vi "S101_ACT2ndCtrl.vi"(0 "SI101_AverageReactorCoolantTemperature.lvclass":refnum<class "SI101_AverageReactorCoolantTemperature.lvclass">, 1 "ACT Loop1":dbl, 2 "ACT Loop2":dbl, 3 "ACT Loop3":dbl, 4 "ACT Loop4":dbl, 5 "error in (no error)":errorcluster, 8 "APs":cluster{"AP1":dbl, "AP2":dbl, "AP3":dbl}) -> (14 "SI101_AverageReactorCoolantTemperature.lvclass out":refnum<class "SI101_AverageReactorCoolantTemperature.lvclass">, 15 "ACT 2nd Ctrl":dbl, 16 "ACT D-Comp":dbl, 17 "ACT 2ND MAX LIM":dbl, 19 "error IO":errorcluster)   [LabVIEW 2022 SP3, in "SI101_AverageReactorCoolantTemperature.lvclass"]
uses:
  SI101_AverageReactorCoolantTemperature.lvclass
  SI101_AverageReactorCoolantTemperature.lvclass/SI101_AverageReactorCoolantTemperature.ctl
panel:
  # "SI101"
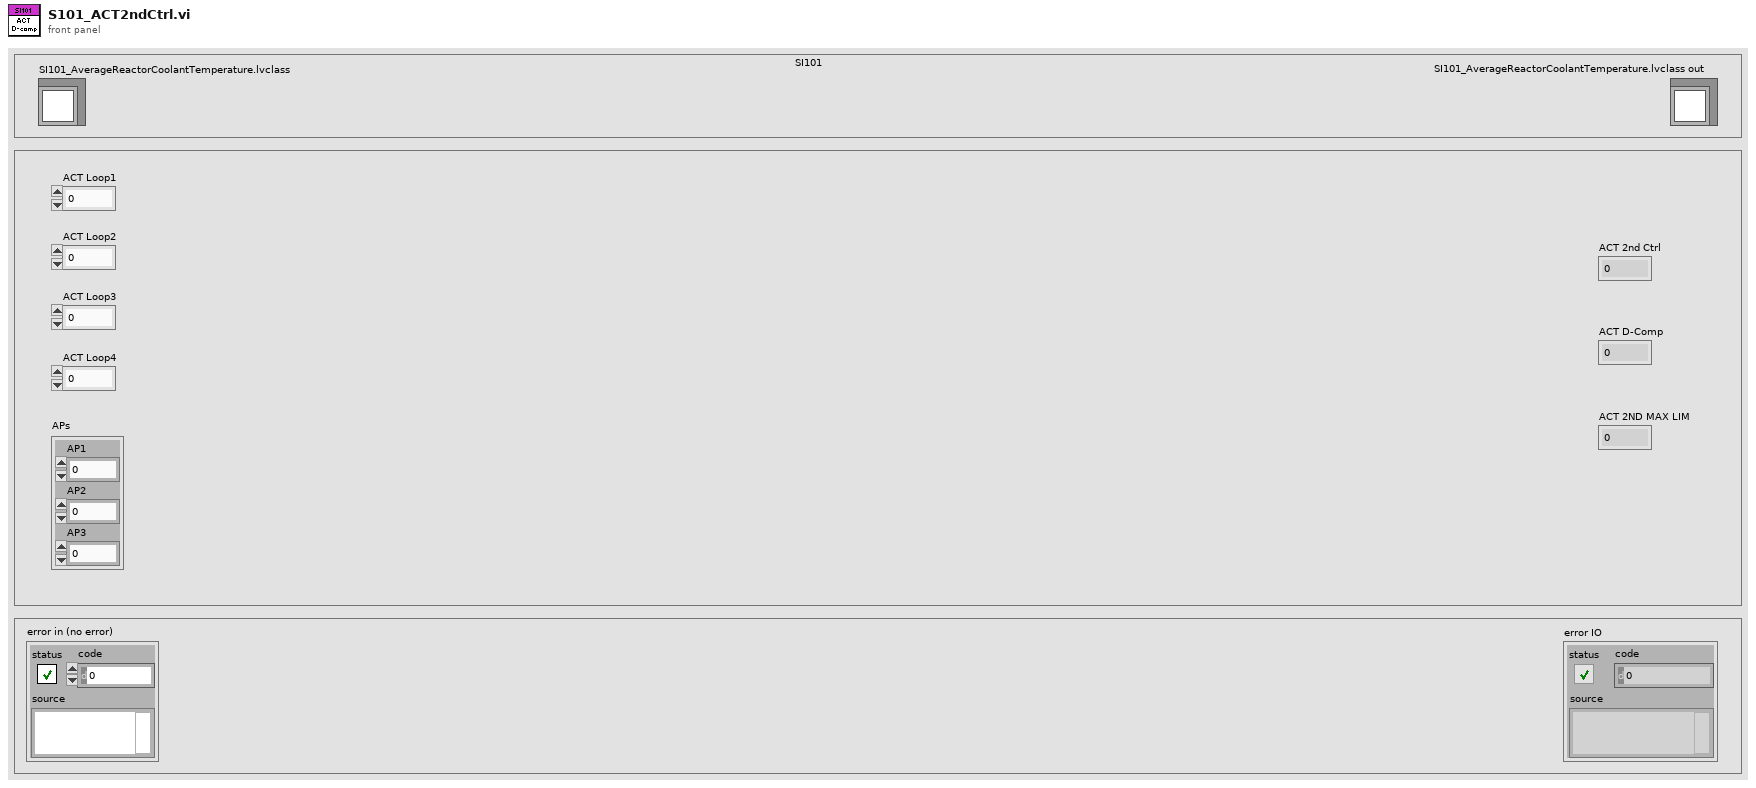
[diagram p1: front panel]
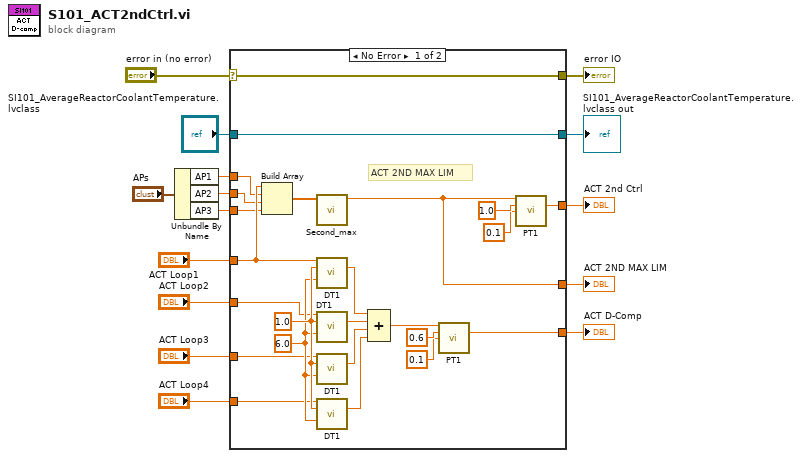
[diagram p0: block diagram]
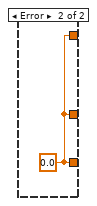
[diagram p2: hidden frame]
diagram:
  n1 = Unbundle By Name("APs") -> ("AP1"=w5:dbl, "AP2"=w4:dbl, "AP3"=w3:dbl)
  n2 = case shown="No Error" "error in (no error)" {
    selector: "error in (no error)" -> [w27 _]
    tunnel: [w31 w40] -> w14
    tunnel: [w28 w40] -> w13
    tunnel: "SI101_AverageReactorCoolantTemperature.lvclass" -> [w18 _]
    tunnel: [w27 _] -> w11
    tunnel: "ACT Loop1" -> [w23 _]
    tunnel: "ACT Loop2" -> [w26 _]
    tunnel: "ACT Loop3" -> [w25 _]
    tunnel: "ACT Loop4" -> [w24 _]
    tunnel: w5 -> [w22 _]
    tunnel: w4 -> [w21 _]
    tunnel: w3 -> [w20 _]
    tunnel: [w18 _] -> w2
    tunnel: [w16 w40] -> w1
    frame No Error {
      w38 = 6.0 ("T1")
      w39 = 1.0 ("G")
      # "ACT 2ND MAX LIM"
      n3 = Build Array(w23, w22, w21, w20) -> (w19:dbl[])
      n4 = call "Second_max.vi"("Array"=w19) -> ("AP3"=w16:dbl)  [unwired: 10 in]
      n5 = call "DT1.vi"("input u(k)"=w23, "G"=w39, "T1"=w38) -> ("output y(k)"=w37:dbl)  [unwired: 11 in, 1 out]
      n6 = call "DT1.vi"("input u(k)"=w26, "G"=w39, "T1"=w38) -> ("output y(k)"=w36:dbl)  [unwired: 11 in, 1 out]
      n7 = call "DT1.vi"("input u(k)"=w25, "G"=w39, "T1"=w38) -> ("output y(k)"=w35:dbl)  [unwired: 11 in, 1 out]
      n8 = call "DT1.vi"("input u(k)"=w24, "G"=w39, "T1"=w38) -> ("output y(k)"=w34:dbl)  [unwired: 11 in, 1 out]
      n9 = Compound Arithmetic op=ADD(w37, w36, w35, w34) -> (w17:dbl)
      n10 = call "PT1.vi"("input u(k)"=w17, "G"=0.6, "T1"=0.1) -> ("output y(k)"=w31:dbl)  [unwired: 11 in, 1 out]
      n11 = call "PT1.vi"("input u(k)"=w16, "G"=1.0, "T1"=0.1) -> ("output y(k)"=w28:dbl)  [unwired: 11 in, 1 out]
    }
    frame Error {
      w40 = 0.0 ("output y(k)")
    }
  }
  "ACT D-Comp" <- w14
  "ACT 2nd Ctrl" <- w13
  "SI101_AverageReactorCoolantTemperature.lvclass out" <- w2
  "error IO" <- w11
  "ACT 2ND MAX LIM" <- w1
